vi "case_structure.vi"() -> ()   [LabVIEW 2020]
panel:
  out "square root":dbl
  in  "input":dbl
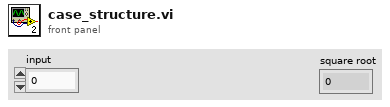
[diagram p1: front panel]
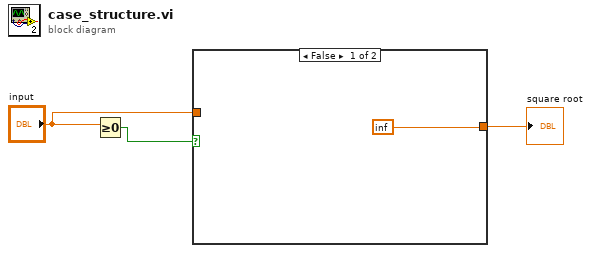
[diagram p0: block diagram]
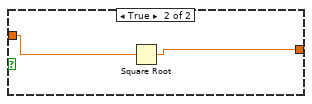
[diagram p2: hidden frame]
diagram:
  n1 = Greater Or Equal To 0?(x="input") -> (x >= 0?=w3:bool)
  n2 = case shown="False" w3 {
    tunnel: "input" -> [_ w6]
    tunnel: [inf w5] -> w1
    frame False {
    }
    frame True {
      n3 = Square Root(x=w6) -> (sqrt(x)=w5:dbl)
    }
  }
  "square root" <- w1
